vi "init.vi"() -> (0 "error out":errorcluster, 3 "Modules":T1)   [LabVIEW 2025]
uses:
  <vilib>/Utility/sysdir.llb/System Directory Type.ctl
  Libraries/USB IO/USB IO.lvlib
  Libraries/Power Supply/Power Supply.lvlib
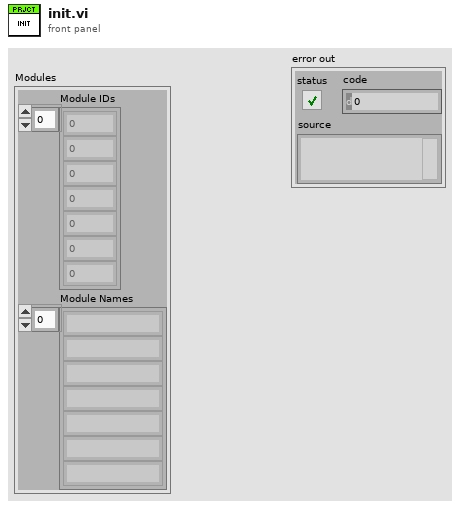
[diagram p1: front panel]
types:
  T1 = cluster{"Module IDs":i32[], "Module Names":string[]}
  T2 = typedef "System Directory Type.ctl" = i32
  T3 = typedef "Hardware Selection.ctl" = enum16{"Simulation", "USB-6000", "USB-6001", "Arduino Uno"}
  T4 = typedef "hardware-selection.ctl" = enum16{"Parent", "Simulation", "PSP-603"}
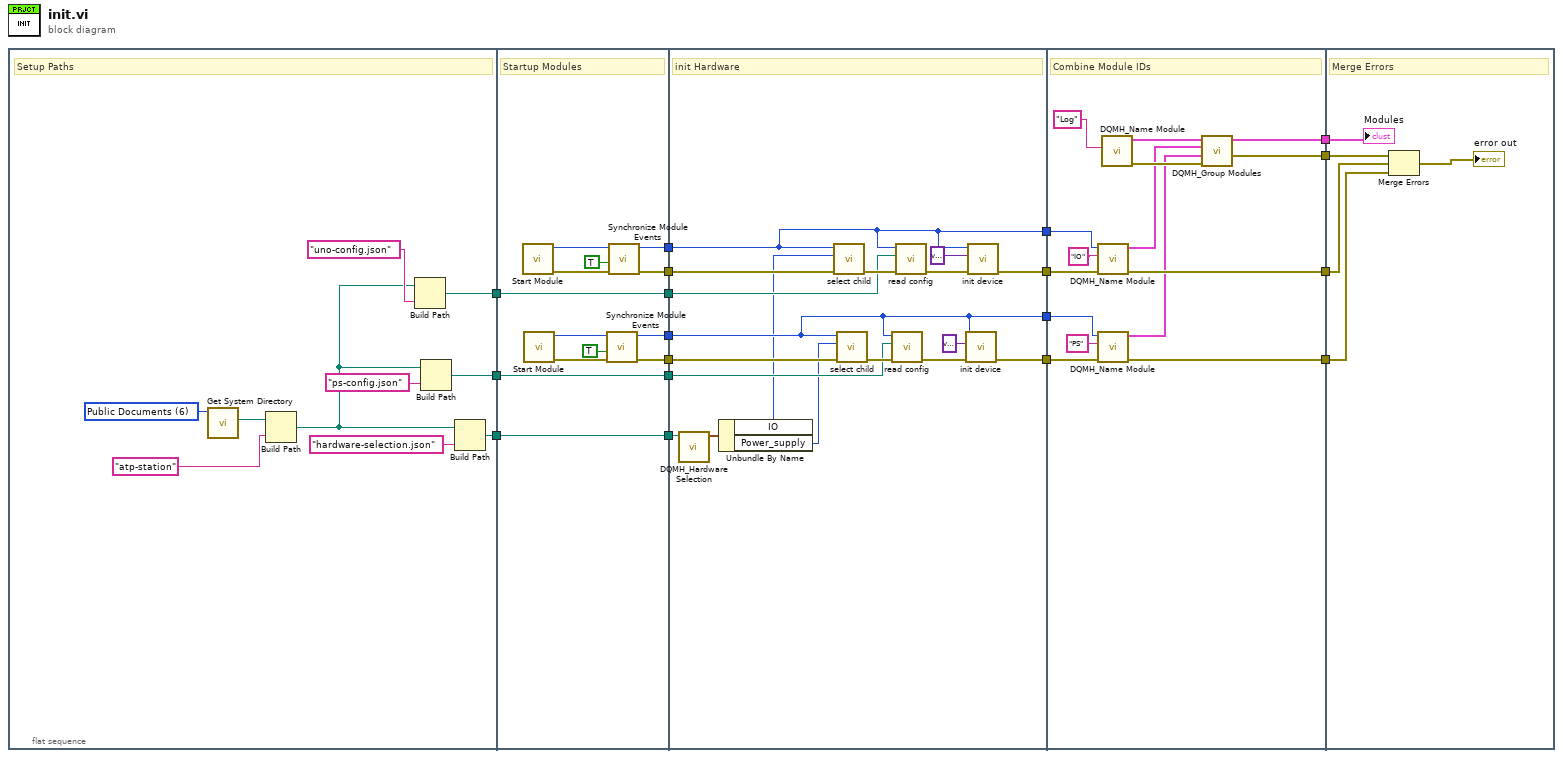
[diagram p0: block diagram]
diagram:
  n1 = flat-sequence {
    tunnel: [w24] -> w14
    tunnel: [w22] -> w8
    tunnel: [w19] -> w2
    tunnel: [w38] -> w16
    tunnel: [w37] -> w15
    tunnel: w14 -> [w36]
    tunnel: [w36] -> w13
    tunnel: [w32] -> w9
    tunnel: w8 -> [w32]
    tunnel: [w31] -> w7
    tunnel: [w30] -> w6
    tunnel: w2 -> [w29]
    tunnel: [w29] -> w1
    tunnel: w16 -> [w54]
    tunnel: w15 -> [w59]
    tunnel: w13 -> [w57]
    tunnel: [w54] -> w12
    tunnel: [w53] -> w11
    tunnel: w9 -> [w50]
    tunnel: w7 -> [w47]
    tunnel: w6 -> [w52]
    tunnel: [w47] -> w5
    tunnel: [w46] -> w4
    tunnel: w1 -> [w45]
    tunnel: [w71] -> w18
    tunnel: [w70] -> w17
    tunnel: w12 -> [w69]
    tunnel: w11 -> [w67]
    tunnel: [w65] -> w10
    tunnel: w5 -> [w64]
    tunnel: w4 -> [w63]
    tunnel: [w60] -> w3
    tunnel: w18 -> [w78]
    tunnel: w17 -> [w79]
    tunnel: w10 -> [w76]
    tunnel: w3 -> [w75]
    frame #0 {
      w28 = T2 6 items=["User Home"=0, "User Desktop"=1, "User Documents"=2, "User Application Data"=3, "User Preferences"=4, "User Temporary"=5, "Public Documents"=6, "Public Application Data"=7, "Public Preferences"=8, "Public Cache"=13, "System Core Libraries"=9, "System Installed Libraries"=10, "Application Files"=11, "Boot Volume Root"=12] ("system directory type")
      # "Setup Paths"
      n2 = call <vilib>:"Get System Directory.vi"("system directory type"=w28) -> ("system directory"=w27:path)  [unwired: 10 in]
      n3 = Build Path(base path=w27, name or relative path="atp-station") -> (appended path=w21:path)
      n4 = Build Path(base path=w21, name or relative path="uno-config.json") -> (appended path=w24:path)
      n5 = Build Path(base path=w21, name or relative path="ps-config.json") -> (appended path=w22:path)
      n6 = Build Path(base path=w21, name or relative path="hardware-selection.json") -> (appended path=w19:path)
    }
    frame #1 {
      # "Startup Modules"
      n7 = call "Start Module.vi"() -> ("error out"=w40:errorcluster, "Module ID"=w41:i32)  [unwired: 7 in, 3 out]
      n8 = call "Start Module.vi"() -> ("error out"=w34:errorcluster, "Module ID"=w35:i32)  [unwired: 7 in, 3 out]
      n9 = call "Synchronize Module Events.vi"("error in"=w34, "Wait for Event Sync?"=TRUE, "Module ID in"=w35) -> ("error out"=w30:errorcluster, "Module ID out"=w31:i32)  [unwired: 7 in]
      n10 = call "Synchronize Module Events.vi"("error in"=w40, "Wait for Event Sync?"=TRUE, "Module ID in"=w41) -> ("error out"=w37:errorcluster, "Module ID out"=w38:i32)  [unwired: 7 in]
    }
    frame #2 {
      # "init Hardware"
      n11 = call "DQMH_Hardware Selection.vi"("File Path"=w45) -> ("Data out"=w44:cluster{"IO":T3, "Power_supply":T4})  [unwired: 10 in]
      n12 = Unbundle By Name(w44) -> ("IO"=w43:T3, "Power_supply"=w42:T4)
      n13 = call "select child.vi"("error in"=w59, "Hardware"=w43, "Module ID"=w54) -> ("error out"=w58:errorcluster)  [unwired: 7 in, 1 out]
      n14 = call "select child.vi"("error in"=w52, "Enum"=w42, "Module ID"=w47) -> ("error out"=w51:errorcluster)  [unwired: 7 in, 1 out]
      n15 = call "read config.vi"("error in"=w51, "config json file"=w50, "Module ID"=w47) -> ("error out"=w49:errorcluster)  [unwired: 7 in, 1 out]
      n16 = call "read config.vi"("error in"=w58, "Path"=w57, "Module ID"=w54) -> ("error out"=w56:errorcluster)  [unwired: 7 in, 1 out]
      n17 = call "init device.vi"("error in"=w49, "Variant"=variant, "Module ID"=w47) -> ("error out"=w46:errorcluster)  [unwired: 7 in, 1 out]
      n18 = call "init device.vi"("error in"=w56, "Variant"=variant, "Module ID"=w54) -> ("error out"=w53:errorcluster)  [unwired: 7 in, 1 out]
    }
    frame #3 {
      # "Combine Module IDs"
      n19 = call "DQMH_Name Module.vi"("error in"=w67, "String"="IO", "Module ID in"=w69) -> ("error out"=w65:errorcluster, "input cluster"=w66:T1)  [unwired: 7 in]
      n20 = call "DQMH_Name Module.vi"("error in"=w63, "String"="PS", "Module ID in"=w64) -> ("error out"=w60:errorcluster, "input cluster"=w61:T1)  [unwired: 7 in]
      n21 = call "DQMH_Name Module.vi"("String"="Log") -> ("error out"=w72:errorcluster, "input cluster"=w73:T1)  [unwired: 9 in]
      n22 = call "DQMH_Group Modules.vi"("error in (no error)"=w72, "Module 3"=w61, "Module 2"=w66, "Module 1"=w73) -> ("error out"=w71:errorcluster, "Modules"=w70:T1)  [unwired: 6 in]
    }
    frame #4 {
      # "Merge Errors"
      n23 = Merge Errors(w78, w76, w75) -> (→"error out":errorcluster)
      "Modules" <- w79
    }
  }
